vi "MGCC_StaEst_complex2magnitude.vi"(10 "st_MGCC_StaEst_Input":T1) -> (2 "output cluster":T1)   [LabVIEW 2016]
uses:
  Model Management/Global_MdlMgmt.vi
  MGCC_StaEst_global.vi
  Communication/Global communication.vi
  <vilib>/imath/engines/lvmath2/RunTimeEngine/IndexRead/NIMS M($,S).vi
  <instcachedir>/0/NIMS M($,S)_3E5749BBB62E49528D4765A77F1F6D98.lvgen/NIMS M($,S)_3E5749BBB62E49528D4765A77F1F6D98_000.vi
  <vilib>/imath/engines/lvmath2/RunTimeEngine/BuiltInFunctions/length/NIMS_length(GV).vi
  <instcachedir>/0/NIMS_length(GV)_08A3D13377FD4E4B96F5795FBF3698FA.lvgen/NIMS_length(GV)_08A3D13377FD4E4B96F5795FBF3698FA_000.vi
  <vilib>/imathl/engines/lvmath/Functions/Error Handling/Create Error.vi
  <vilib>/imath/engines/lvmath2/RunTimeEngine/RangeToken/NIMS_Range_R3 - Integer.vi
  <instcachedir>/0/NIMS_Range_R3 - Integer_A435E2FF893B4C718FD5055FE39FE2F6.lvgen/NIMS_Range_R3 - Integer_A435E2FF893B4C718FD5055FE39FE2F6_000.vi
  <vilib>/imath/engines/lvmath2/RunTimeEngine/CommandStatement/MC_CommandStatement_break.vi
  <vilib>/imath/engines/lvmath2/RunTimeEngine/BuiltInFunctions/findnz/NIMS_[1o]_findnz(GRowV).vi
  <instcachedir>/0/NIMS_[1o]_findnz(GRowV)_1AF74843B4874134ADE908C0A4A72F3C.lvgen/NIMS_[1o]_findnz(GRowV)_1AF74843B4874134ADE908C0A4A72F3C_000.vi
  <vilib>/imath/engines/lvmath2/RunTimeEngine/BuiltInFunctions/is_empty/NIMS_is_empty(GV).vi
  <instcachedir>/0/NIMS_is_empty(GV)_FC7E7C3D9544432CB6AA2416ADCF6D56.lvgen/NIMS_is_empty(GV)_FC7E7C3D9544432CB6AA2416ADCF6D56_000.vi
  <vilib>/imath/engines/lvmath2/RunTimeEngine/IndexRead/NIMS M(S,S).vi
  <instcachedir>/0/NIMS M(S,S)_AC51E74150A542F7991B9634C66F3096.lvgen/NIMS M(S,S)_AC51E74150A542F7991B9634C66F3096_000.vi
  <vilib>/imath/engines/lvmath2/RunTimeSupport/NIMS_Error if Not Equal.vi
  <instcachedir>/0/NIMS_Error if Not Equal_43252A79AD05436189442EC0C5E5AB8A.lvgen/NIMS_Error if Not Equal_43252A79AD05436189442EC0C5E5AB8A_000.vi
  <vilib>/imath/engines/lvmath2/RunTimeEngine/IndexRead/NIMS V(S).vi
  <instcachedir>/0/NIMS V(S)_0488751826AF41519A22953C041130DC.lvgen/NIMS V(S)_0488751826AF41519A22953C041130DC_000.vi
  <vilib>/imath/engines/lvmath2/RunTimeEngine/IndexReplace/NIMS M(S,S)=S.vi
  <instcachedir>/0/NIMS M(S,S)=S_98E40400474E4398B113AE20298B4F82.lvgen/NIMS M(S,S)=S_98E40400474E4398B113AE20298B4F82_000.vi
  <vilib>/imath/engines/lvmath2/RunTimeEngine/ErrorHandling/NIMS_Create Error From Enums.vi
  <vilib>/imath/engines/lvmath2/RunTimeEngine/NodeEndStatement/NIMS_NodeEndStatement_Output.vi
  <instcachedir>/0/NIMS_NodeEndStatement_Output_53EC0D466D134D7ABD903AC30B43404B.lvgen/NIMS_NodeEndStatement_Output_53EC0D466D134D7ABD903AC30B43404B_002.vi
  <vilib>/imath/engines/lvmath2/RunTimeEngine/ErrorHandling/NIMS_Finalize Error.vi
  <vilib>/Utility/error.llb/Error Cluster From Error Code.vi
  <vilib>/ErrorRing/Error Ring.xnode
panel:
  out "error out":errorcluster
  out "appended array":dbl[][](array[numeric])
  out "V_node":cdb[][](array[numeric])
  out "r * e^(i*theta)":cdb[][](array[numeric])
  out "output array":dbl[][](array[numeric])
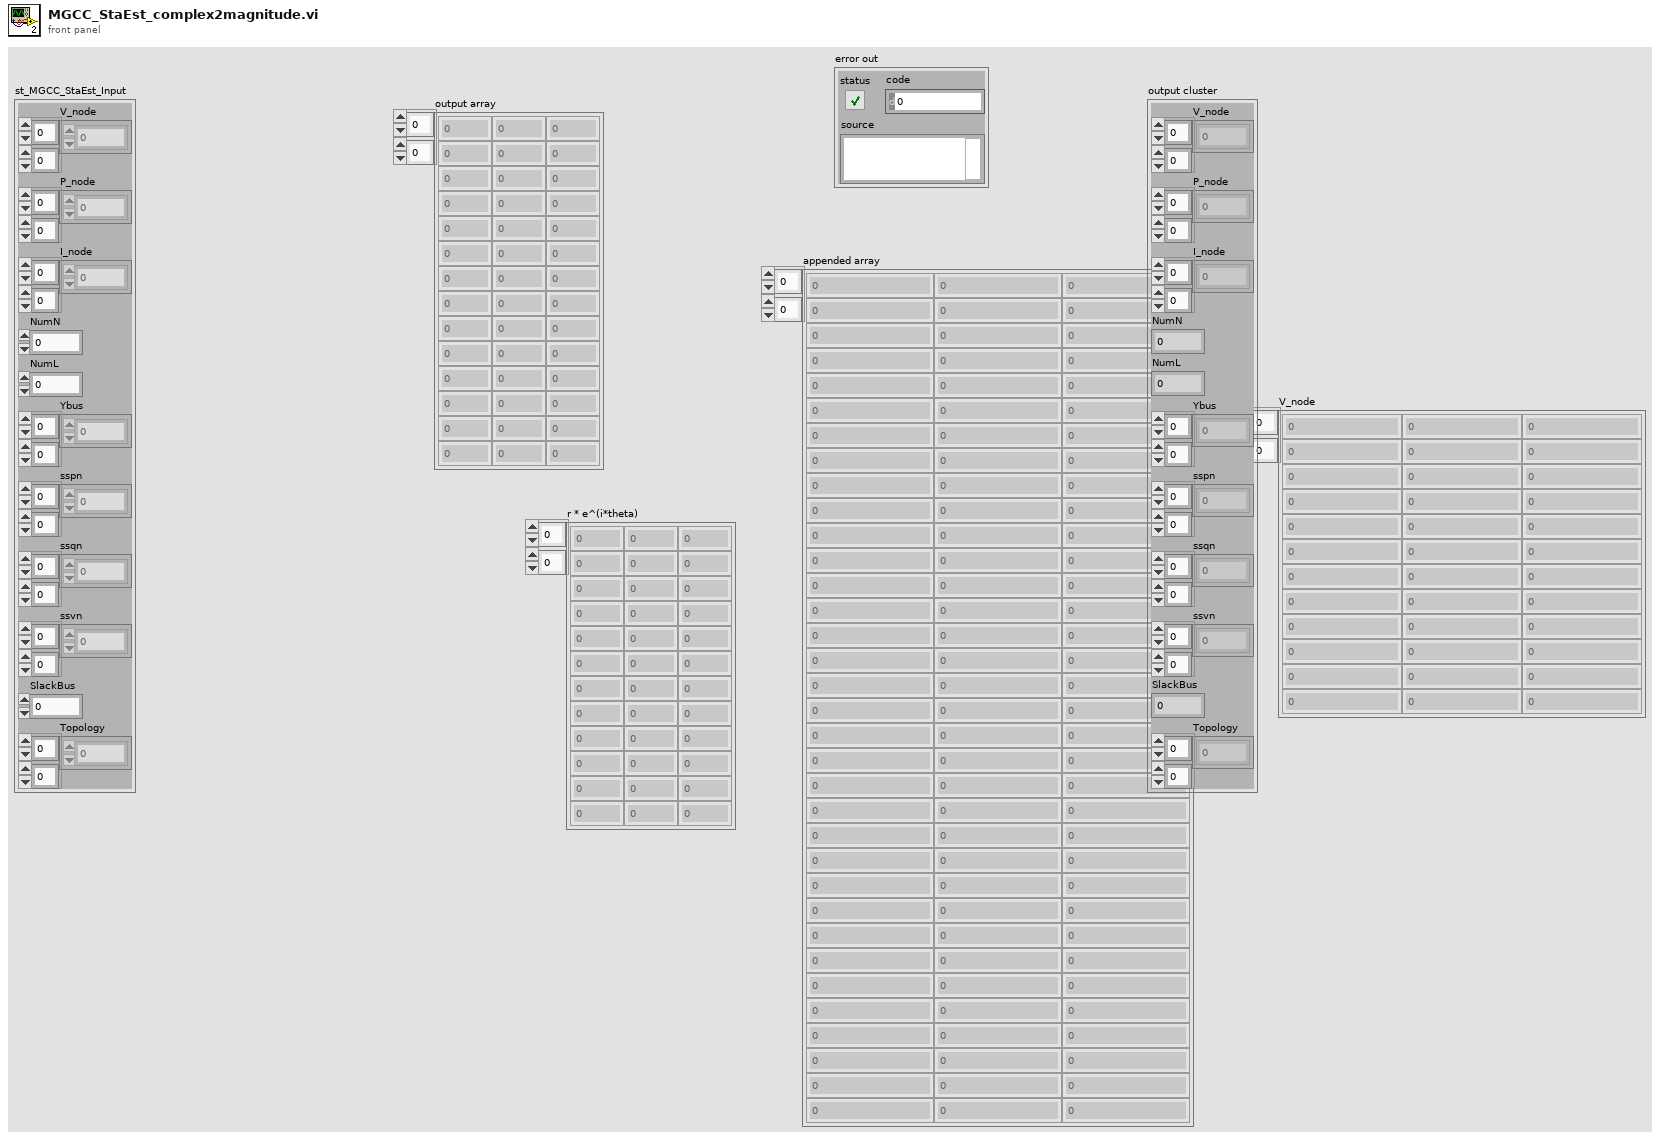
[diagram p1: front panel]
types:
  T1 = cluster{"V_node":cdb[][], "P_node":cdb[][], "I_node":cdb[][], "NumN":dbl, "NumL":dbl, "Ybus":cdb[][], "sspn":dbl[][], "ssqn":dbl[][], "ssvn":dbl[][], "SlackBus":dbl, "Topology":dbl[][]}
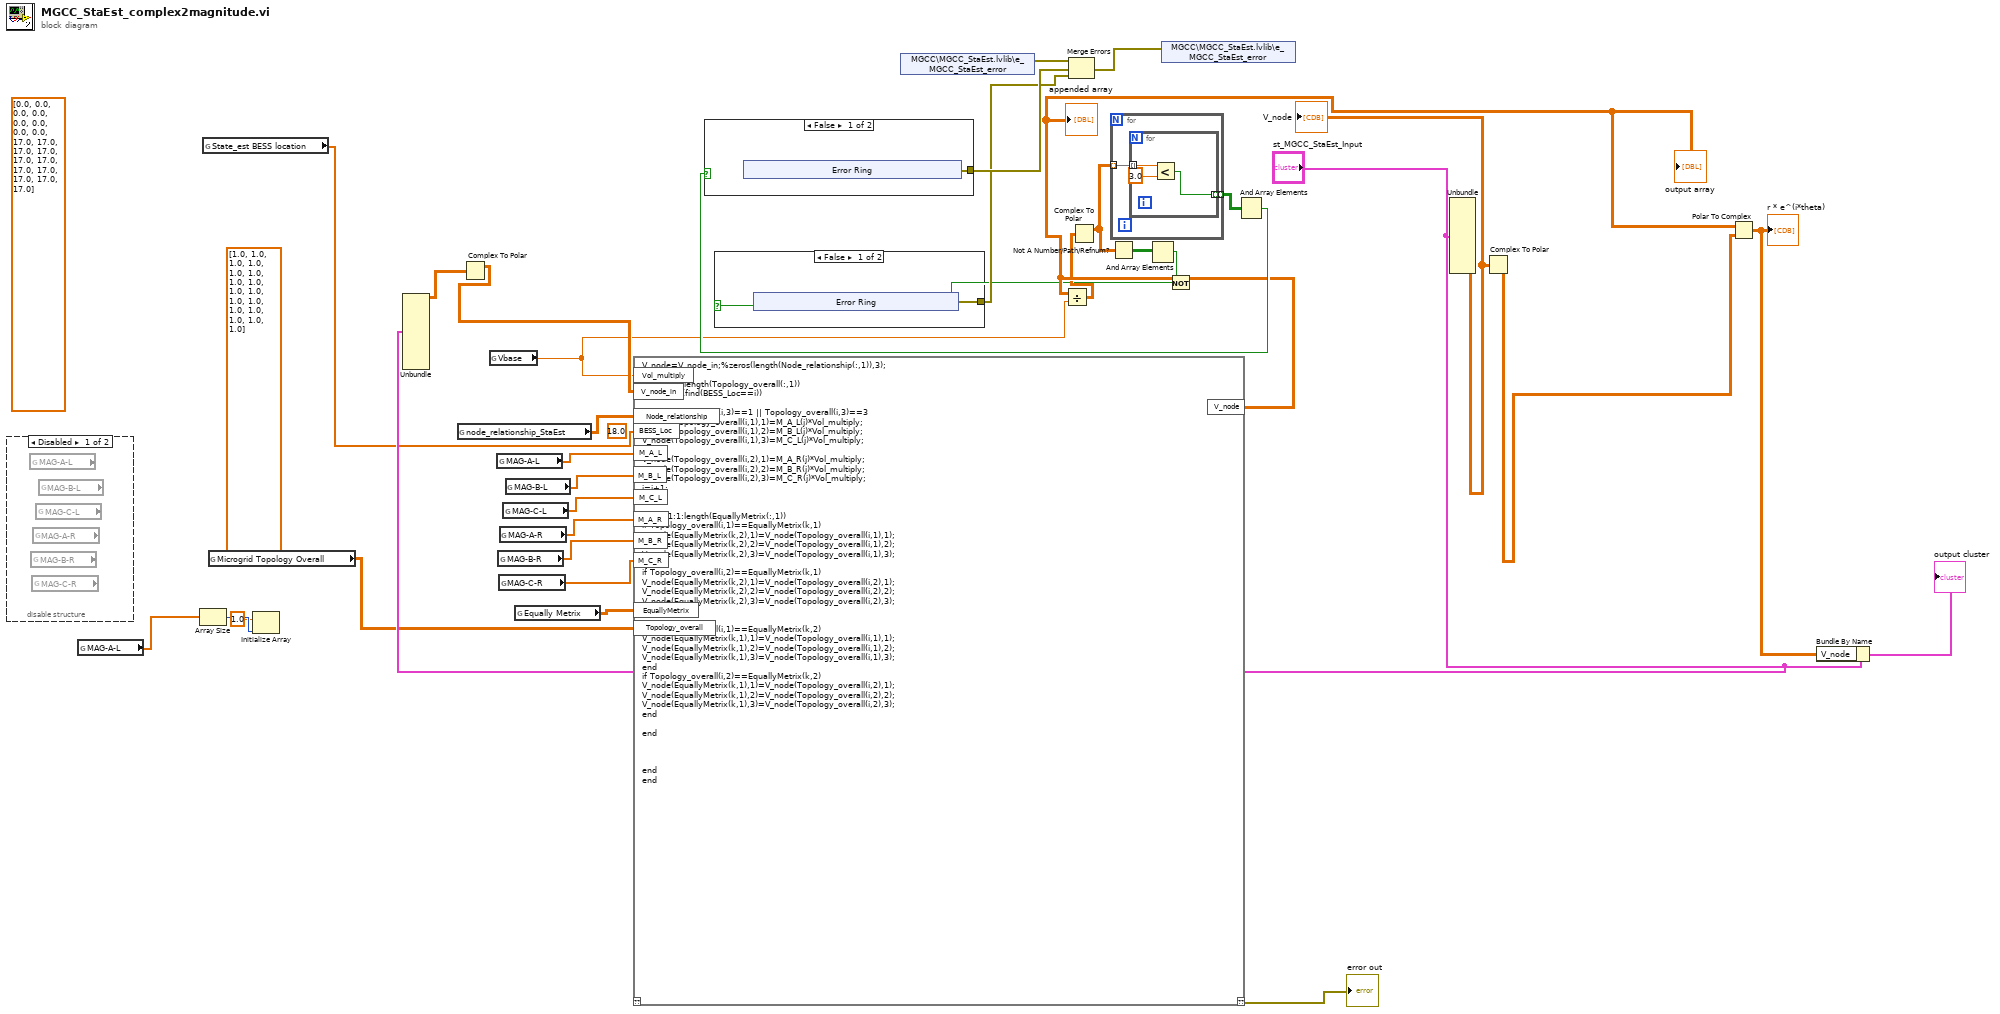
[diagram p0: block diagram]
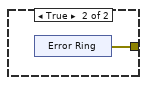
[diagram p3: hidden frame]
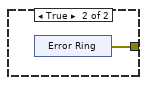
[diagram p4: hidden frame]
diagram:
  (unwired) dbl[] [1.0, 1.0, 1.0, 1.0, 1.0, 1.0, 1.0, 1.0, 1.0, 1.0, 1.0, 1.0, 1.0, 1.0, 1.0, 1.0, 1.0] ("Load_active")
  (unwired) dbl[] [0.0, 0.0, 0.0, 0.0, 0.0, 0.0, 0.0, 0.0, 17.0, 17.0, 17.0, 17.0, 17.0, 17.0, 17.0, 17.0, 17.0, 17.0, 17.0] ("Load_active")
  (unwired) 18.0 ("BESS_Loc")
  n1 = disable-structure shown="Disabled" {
    frame Disabled {
      n2 = global read "Global communication.vi" "MAG-A-L"() -> (w39:dbl[])
      n3 = global read "Global communication.vi" "MAG-B-R"() -> (w35:dbl[])
      n4 = global read "Global communication.vi" "MAG-C-R"() -> ()  [unwired: 1 out]
      n5 = global read "Global communication.vi" "MAG-A-R"() -> (w36:dbl[])
      n6 = global read "Global communication.vi" "MAG-C-L"() -> (w37:dbl[])
      n7 = global read "Global communication.vi" "MAG-B-L"() -> (w38:dbl[])
    }
    frame Enabled {
    }
  }
  n8 = global read "Global communication.vi" "MAG-A-L"() -> (w9:dbl[])
  n9 = Array Size(array=w9) -> (size(s)=w8:i32)
  n10 = global read "Global_MdlMgmt.vi" "State_est BESS location"() -> (w11:dbl[])
  n11 = global read "Global_MdlMgmt.vi" "Microgrid Topology Overall"() -> (w25:dbl[][])
  n12 = Initialize Array(1.0 ("element"), w8) -> ()  [unwired: 1 out]
  n13 = Unbundle("st_MGCC_StaEst_Input") -> ("V_node"=w30:cdb[][])  [unwired: 10 out]
  n14 = global read "Global_MdlMgmt.vi" "node_relationship_StaEst"() -> (w29:dbl[][])
  n15 = Complex To Polar(r * e^(i*theta)=w30) -> (r=w28:dbl[][])  [unwired: 1 out]
  n16 = global read "MGCC_StaEst_global.vi" "Vbase"() -> (w10:dbl)
  n17 = global read "Global communication.vi" "MAG-A-L"() -> (w6:dbl[])
  n18 = global read "Global communication.vi" "MAG-B-R"() -> (w2:dbl[])
  n19 = global read "Global communication.vi" "MAG-C-R"() -> (w1:dbl[])
  n20 = global read "Global communication.vi" "MAG-A-R"() -> (w3:dbl[])
  n21 = global read "Global communication.vi" "MAG-C-L"() -> (w4:dbl[])
  n22 = global read "Global communication.vi" "MAG-B-L"() -> (w5:dbl[])
  n23 = global read "Global_MdlMgmt.vi" "Equally Metrix"() -> (w26:dbl[][])
  n24 = mathscript code="V_node=V_node_in;%zeros(length(Node_relationship(:,1)),3);\nj=1;\nfor i =1:1:length(Topology_overall(:,1))\nif isempty(find(BESS_Loc==i))\n\nif Topology_overall(i,3)==1 || Topology_overall(i,3)==3\nV_node(Topology_overall(i,1),1)=M_A_L(j)*Vol_multiply;\nV_node(Topology_overall(i,1),2)=M_B_L(j)*Vol_multiply;\nV_node(Topology_overall(i,1),3)=M_C_L(j)*Vol_multiply;\n\nV_node(Topology_overall(i,2),1)=M_A_R(j)*Vol_multiply;\nV_node(Topology_overall(i,2),2)=M_B_R(j)*Vol_multiply;\nV_node(Topology_overall(i,2),3)=M_C_R(j)*Vol_multiply;\nj=j+1;\nend\n\nfor k=1:1:length(EquallyMetrix(:,1))\nif Topology_overall(i,1)==EquallyMetrix(k,1)\nV_node(EquallyMetrix(k,2),1)=V_node(Topology_overall(i,1),1);\nV_node(EquallyMetrix(k,2),2)=V_node(Topology_overall(i,1),2);\nV_node(EquallyMetrix(k,2),3)=V_node(Topology_overall(i,1),3);\nend\nif Topology_overall(i,2)==EquallyMetrix(k,1)\nV_node(EquallyMetrix(k,2),1)=V_node(Topology_overall(i,2),1);\nV_node(EquallyMetrix(k,2),2)=V_node(Topology_overall(i,2),2);\nV_node(EquallyMetrix(k,2),3)=V_node(Topology_overall(i,2),3);\nend\n\nif Topology_overall(i,1)==EquallyMetrix(k,2)\nV_node(EquallyMetrix(k,1),1)=V_node(Topology_overall(i,1),1);\nV_node(EquallyMetrix(k,1),2)=V_node(Topology_overall(i,1),2);\nV_node(EquallyMetrix(k,1),3)=V_node(Topology_overall(i,1),3);\nend\nif Topology_overall(i,2)==EquallyMetrix(k,2)\nV_node(EquallyMetrix(k,1),1)=V_node(Topology_overall(i,2),1);\nV_node(EquallyMetrix(k,1),2)=V_node(Topology_overall(i,2),2);\nV_node(EquallyMetrix(k,1),3)=V_node(Topology_overall(i,2),3);\nend\n\nend\n\n\n\nend\nend"("Node_relationship"=w29, "Vol_multiply"=w10, "M_A_L"=w6, "M_B_L"=w5, "M_C_L"=w4, "M_A_R"=w3, "M_B_R"=w2, "M_C_R"=w1, "V_node_in"=w28, "BESS_Loc"=w11, "EquallyMetrix"=w26, "Topology_overall"=w25) -> ("??"=→"error out":errorcluster, "V_node"=w14:dbl[][])  [unwired: 1 in]
  "output array" <- w14
  "appended array" <- w14
  n25 = shared-variable "MGCC\\MGCC_StaEst.lvlib\\e_MGCC_StaEst_error"() -> (w24:errorcluster)  [unwired: 1 in, 1 out]
  n26 = Divide(x=w14, y=w10) -> (x/y=w13:dbl[][])
  n27 = Complex To Polar(r * e^(i*theta)=w13) -> (r=w18:dbl[][])  [unwired: 1 out]
  n28 = for {
    tunnel: w18 -> [w41] mode=indexing
    tunnel: [w40] -> w17 mode=indexing
    n29 = for {
      tunnel: w41 -> [w44] mode=indexing
      tunnel: [w42] -> w40 mode=indexing
      n30 = Less?(x=w44, y=3.0) -> (x < y?=w42:bool)
    }
  }
  n31 = Not A Number/Path/Refnum?(number/path/refnum=w18) -> (NaN/Path/Refnum?=w21:bool[][])
  n32 = And Array Elements(Boolean array=w21) -> (logical AND=w20:bool)
  n33 = Not(x=w20) -> (.not. x?=w12:bool)
  n34 = case shown="False" w12 {
    tunnel: [w45 w51] -> w19
    frame False {
      n35 = xnode "Error Ring"() -> ("error out"=w45:errorcluster)
    }
    frame True {
      n36 = xnode "Error Ring"() -> ("error out"=w51:errorcluster)
    }
  }
  n37 = And Array Elements(Boolean array=w17) -> (logical AND=w16:bool)
  n38 = case shown="False" w16 {
    tunnel: [w53 w59] -> w22
    frame False {
      n39 = xnode "Error Ring"() -> ("error out"=w53:errorcluster)
    }
    frame True {
      n40 = xnode "Error Ring"() -> ("error out"=w59:errorcluster)
    }
  }
  n41 = Merge Errors(w24, w22, w19) -> (w23:errorcluster)
  n42 = shared-variable "MGCC\\MGCC_StaEst.lvlib\\e_MGCC_StaEst_error"(w23) -> ()  [unwired: 1 in, 1 out]
  n43 = Unbundle("st_MGCC_StaEst_Input") -> ("V_node"=w32:cdb[][])  [unwired: 10 out]
  "V_node" <- w32
  n44 = Complex To Polar(r * e^(i*theta)=w32) -> (theta=w31:dbl[][])  [unwired: 1 out]
  n45 = Polar To Complex(1:w31, 2:w14) -> (0:w34:cdb[][])
  "r * e^(i*theta)" <- w34
  n46 = Bundle By Name(cluster="st_MGCC_StaEst_Input", "V_node"=w34) -> (→"output cluster":T1)
